vi "SandwitchingValues.vi"(8 "DesiredAngle":dbl, 10 "Angle Array":dbl[](array[numeric])) -> (3 "Angle Indexes":dbl[](array[numeric]))   [LabVIEW 2011, in "LinearInterpolation.lvclass"]
doc: "Determines indecies of angles in the input array sandwitching the desired Array"
uses:
  LinearInterpolation.lvclass
panel:
  out "guessed angle":dbl
  out "bigger than value?":bool
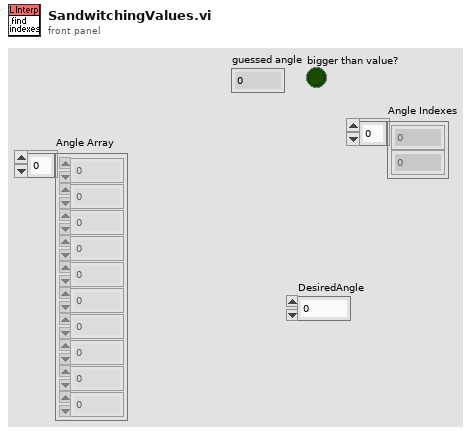
[diagram p1: front panel]
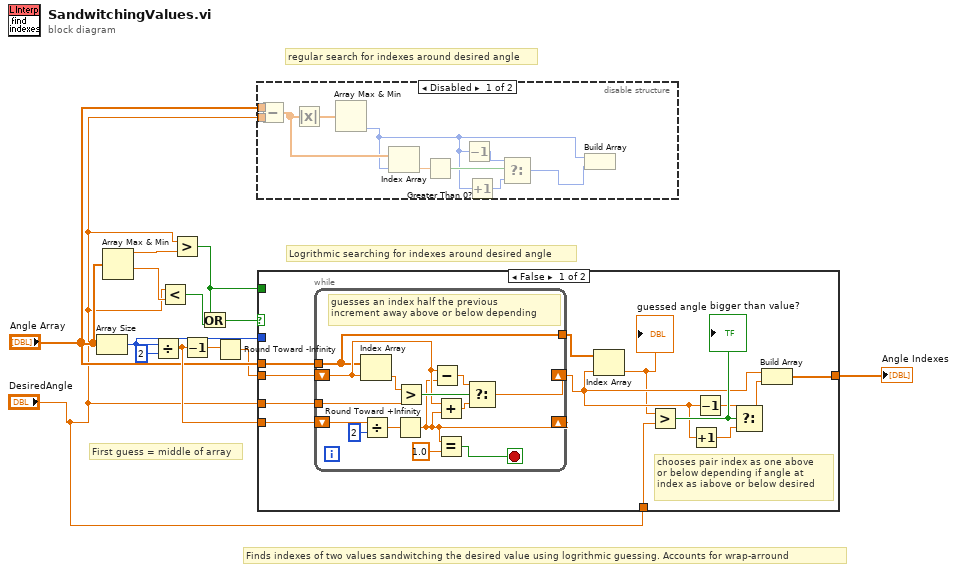
[diagram p0: block diagram]
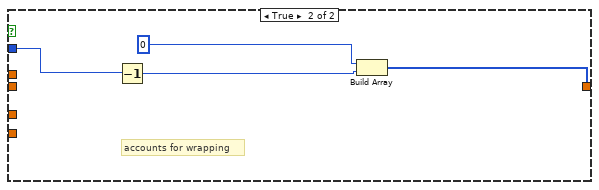
[diagram p2: hidden frame]
diagram:
  # "regular search for indexes around desired angle"
  # "Logrithmic searching for indexes around desired angle"
  # "First guess = middle of array"
  # "Finds indexes of two values sandwitching the desired value using logrithmic guessing. Accounts for wrap-arround"
  n1 = Array Size(array="Angle Array") -> (size(s)=w8:i32)
  n2 = Array Max & Min(array="Angle Array") -> (max value=w4:dbl, min value=w6:dbl)  [unwired: 2 out]
  n3 = Divide(x=w8, y=2) -> (x/y=w12:dbl)
  n4 = Less?(x="DesiredAngle", y=w6) -> (x < y?=w9:bool)
  n5 = Greater?(x="DesiredAngle", y=w4) -> (0:w5:bool)
  n6 = Decrement(x=w12) -> (x-1=w2:dbl)
  n7 = Or(x=w5, y=w9) -> (x .or. y?=w11:bool)
  n8 = Round Toward -Infinity(1:w2) -> (0:w1:dbl)
  n9 = disable-structure shown="Disabled" {
    disable-tunnel: "Angle Array" -> [w15 _]
    disable-tunnel: "DesiredAngle" -> [w14 _]
    frame Disabled {
      n10 = Subtract(x=w15, y=w14) -> (x-y=w23:dbl[])
      n11 = Absolute Value(x=w23) -> (abs(x)=w24:dbl[])
      n12 = Array Max & Min(array=w24) -> (min index (indices)=w18:i32)  [unwired: 3 out]
      n13 = Index Array(array=w23, index=w18) -> (element=w22:dbl)
      n14 = Greater Than 0?(x=w22) -> (x > 0?=w21:bool)
      n15 = Decrement(x=w18) -> (x-1=w19:i32)
      n16 = Increment(x=w18) -> (x+1=w20:i32)
      n17 = Select(t=w19, s=w21, f=w20) -> (s? t:f=w17:i32)
      n18 = Build Array(w18, w17) -> (w16:i32[])
    }
    frame Enabled {
    }
  }
  n19 = case shown="False" w11 {
    tunnel: "Angle Array" -> [w37 _]
    tunnel: w1 -> [w36 _]
    tunnel: w12 -> [w35 _]
    tunnel: "DesiredAngle" -> [w34 _]
    tunnel: [w29 w52] -> w7
    tunnel: w5 -> [_ _]
    tunnel: w8 -> [_ w55]
    tunnel: "DesiredAngle" -> [w25 _]
    frame False {
      # "chooses pair index as one above  \nor below depending if angle at \nindex as iabove or below desired"
      n20 = while {
        tunnel: w37 -> [w38]
        tunnel: w34 -> [w50]
        shift-right: [w45] -> w27
        shift-left: w36 -> [w46]
        shift-right: [w39] -> _
        shift-left: w35 -> [w42]
        tunnel: [w38] -> w28
        stop <- w40 stop-if-true
        # "guesses an index half the previous \nincrement away above or below depending"
        n21 = Index Array(array=w38, index=w46) -> (element=w51:dbl)
        n22 = Divide(x=w42, y=2) -> (x/y=w44:dbl)
        n23 = Round Toward +Infinity(x=w44) -> (ceil(x): smallest int >= x=w39:dbl)
        n24 = Greater?(x=w51, y=w50) -> (0:w49:bool)
        n25 = Subtract(x=w46, y=w39) -> (x-y=w48:dbl)
        n26 = Add(x=w46, y=w39) -> (x+y=w47:dbl)
        n27 = Equal?(x=w39, y=1.0) -> (x = y?=w40:bool)
        n28 = Select(t=w48, s=w49, f=w47) -> (s? t:f=w45:dbl)
      }
      n29 = Index Array(array=w28, index=w27) -> (element=w26:dbl)
      "guessed angle" <- w26
      n30 = Greater?(x=w26, y=w25) -> (0:w33:bool)
      "bigger than value?" <- w33
      n31 = Increment(x=w27) -> (x+1=w31:dbl)
      n32 = Decrement(x=w27) -> (x-1=w32:dbl)
      n33 = Select(t=w32, s=w33, f=w31) -> (s? t:f=w30:dbl)
      n34 = Build Array(w27, w30) -> (w29:dbl[])
    }
    frame True {
      # "accounts for wrapping"
      n35 = Decrement(x=w55) -> (x-1=w53:i32)
      n36 = Build Array(0 ("t"), w53) -> (w52:i32[])
    }
  }
  "Angle Indexes" <- w7
